vi "singleShot_defaultSetup.vi"() -> ()   [LabVIEW 2016]
uses:
  <userlib>/RSA_API/RSA_API.lvlib
panel:
  out "settings out":T1 {"window" items=["SpectrumWindow_Kaiser", "SpectrumWindow_Mil6dB", "SpectrumWindow_BlackmanHarris", "SpectrumWindow_Rectangle", "SpectrumWindow_FlatTop", "SpectrumWindow_Hann"]; "verticalUnit" items=["SpectrumVerticalUnit_dBm", "SpectrumVerticalUnit_Watt", "SpectrumVerticalUnit_Volt", "SpectrumVerticalUnit_Amp", "SpectrumVerticalUnit_dBmV"]}
  in  "Trace number":u32(ring) items=["SpectrumTrace1", "SpectrumTrace2", "SpectrumTrace3"]
  out "traceData out":sgl[](graph)
  out "outTracePoints out":i32
  out "Trace Ready":bool
  out "enable out":bool
  out "refLevel out":dbl
  out "cf out":dbl
  in  "deviceID":i32
  out "deviceType out":string
  out "deviceSerial out":string
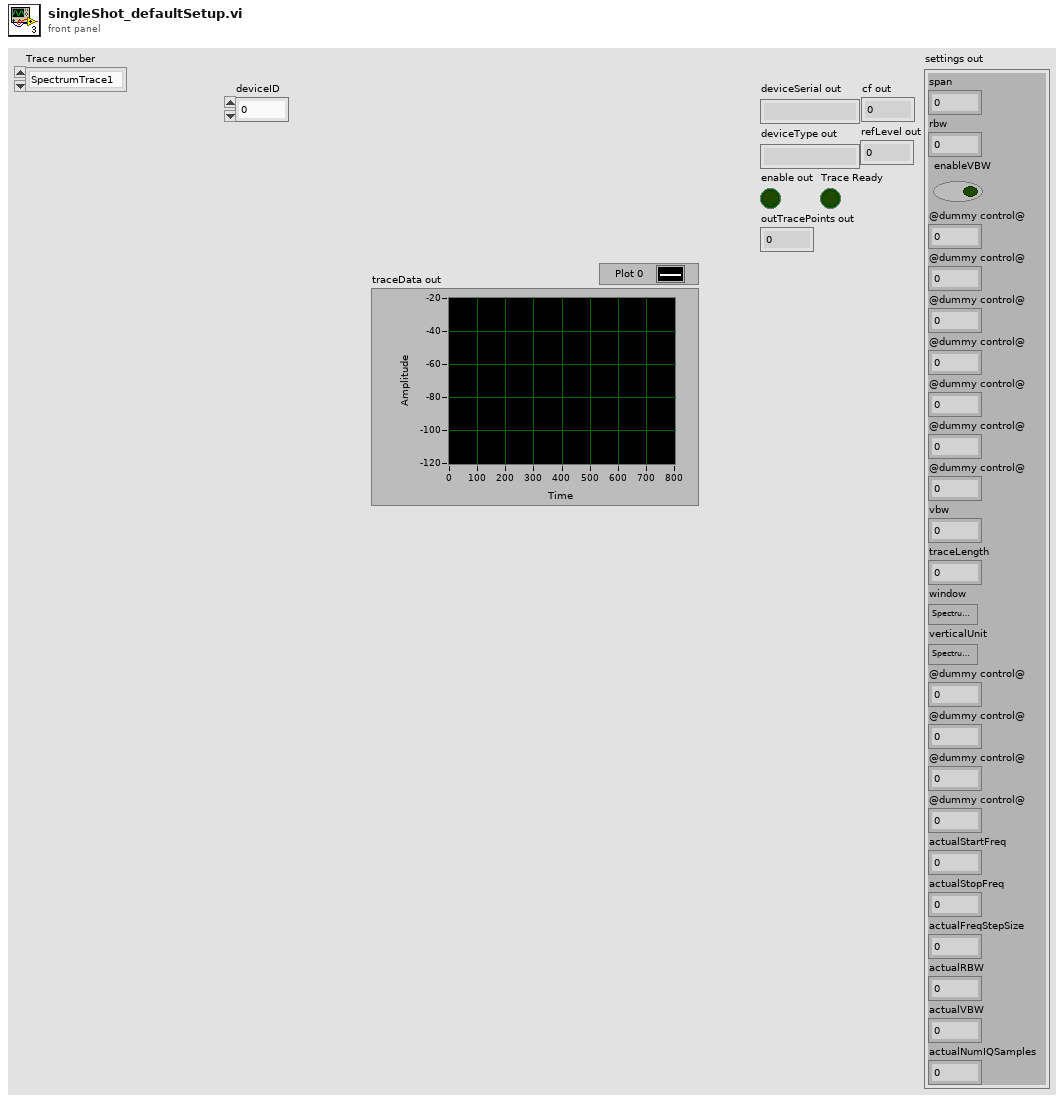
[diagram p1: front panel]
types:
  T1 = cluster{"span":dbl, "rbw":dbl, "enableVBW":bool, "@dummy control@":i8, "@dummy control@":i8, "@dummy control@":i8, "@dummy control@":i8, "@dummy control@":i8, "@dummy control@":i8, "@dummy control@":i8, "vbw":dbl, "traceLength":i32, "window":u32, "verticalUnit":u32, "@dummy control@":i8, "@dummy control@":i8, "@dummy control@":i8, "@dummy control@":i8, "actualStartFreq":dbl, "actualStopFreq":dbl, "actualFreqStepSize":dbl, "actualRBW":dbl, "actualVBW":dbl, "actualNumIQSamples":i32}
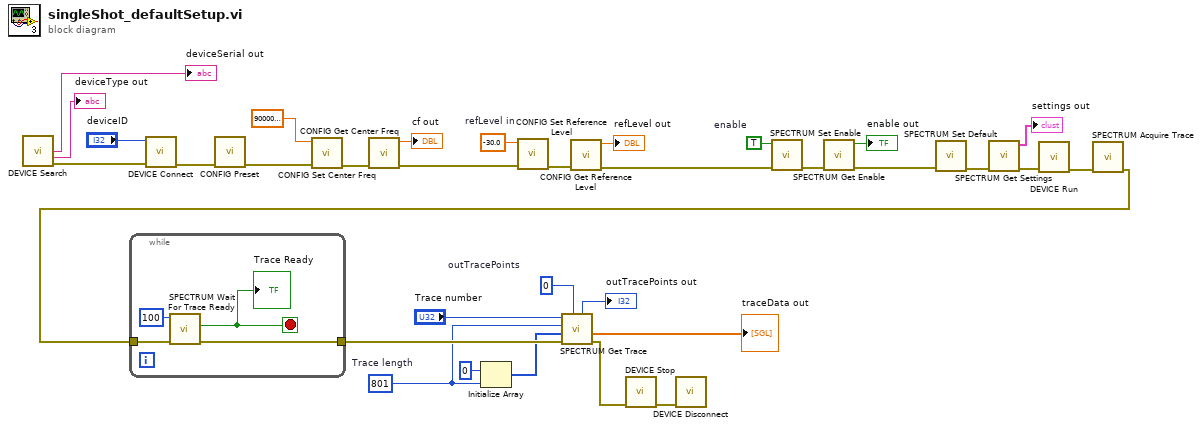
[diagram p0: block diagram]
diagram:
  w19 = TRUE  # enable
  w22 = -30.0  # refLevel in
  w10 = 801  # Trace length
  w11 = 0  # outTracePoints
  n1 = call <userlib>:"DEVICE Search.vi"() -> ("deviceSerial out"=→"deviceSerial out":string, "deviceType out"=→"deviceType out":string, "error out"=w30:errorcluster)  [unwired: 10 in, 3 out]
  n2 = call <userlib>:"DEVICE Connect.vi"("error in (no error)"=w30, "deviceID"="deviceID") -> ("error out"=w29:errorcluster)  [unwired: 8 in, 1 out]
  n3 = call <userlib>:"CONFIG Preset.vi"("error in (no error)"=w29) -> ("error out"=w28:errorcluster)  [unwired: 9 in, 1 out]
  n4 = call <userlib>:"CONFIG Set Center Freq.vi"("error in (no error)"=w28, "cf"=90000000.0) -> ("error out"=w27:errorcluster)  [unwired: 8 in, 1 out]
  n5 = call <userlib>:"CONFIG Get Center Freq.vi"("error in (no error)"=w27) -> ("error out"=w26:errorcluster, "cf out"=→"cf out":dbl)  [unwired: 8 in, 1 out]
  n6 = Initialize Array(0 ("element"), w10) -> (w8:i32[])
  n7 = call <userlib>:"CONFIG Set Reference Level.vi"("error in (no error)"=w26, "refLevel"=w22) -> ("error out"=w25:errorcluster)  [unwired: 8 in, 1 out]
  n8 = call <userlib>:"CONFIG Get Reference Level.vi"("error in (no error)"=w25) -> ("error out"=w20:errorcluster, "refLevel out"=→"refLevel out":dbl)  [unwired: 8 in, 1 out]
  n9 = call <userlib>:"SPECTRUM Set Enable.vi"("error in (no error)"=w20, "enable"=w19) -> ("error out"=w18:errorcluster)  [unwired: 8 in, 1 out]
  n10 = call <userlib>:"SPECTRUM Get Enable.vi"("error in (no error)"=w18) -> ("error out"=w16:errorcluster, "enable out"=→"enable out":bool)  [unwired: 8 in, 1 out]
  n11 = call <userlib>:"SPECTRUM Set Default.vi"("error in (no error)"=w16) -> ("error out"=w3:errorcluster)  [unwired: 9 in, 1 out]
  n12 = call <userlib>:"SPECTRUM Get Settings.vi"("error in (no error)"=w3) -> ("error out"=w2:errorcluster, "settings out"=→"settings out":T1)  [unwired: 8 in, 1 out]
  n13 = call <userlib>:"DEVICE Run.vi"("error in (no error)"=w2) -> ("error out"=w15:errorcluster)  [unwired: 9 in, 1 out]
  n14 = call <userlib>:"SPECTRUM Acquire Trace.vi"("error in (no error)"=w15) -> ("error out"=w14:errorcluster)  [unwired: 9 in, 1 out]
  n15 = while {
    tunnel: w14 -> [w35]
    tunnel: [w34] -> w13
    stop <- w36 stop-if-true
    n16 = call <userlib>:"SPECTRUM Wait For Trace Ready.vi"("error in (no error)"=w35, "timeoutMsec"=100) -> ("error out"=w34:errorcluster, "ready out"=w36:bool)  [unwired: 7 in, 1 out]
    "Trace Ready" <- w36
  }
  n17 = call <userlib>:"SPECTRUM Get Trace.vi"("outTracePoints"=w11, "error in (no error)"=w13, "traceData"=w8, "maxTracePoints"=w10, "trace"="Trace number") -> ("error out"=w5:errorcluster, "traceData out"=→"traceData out":sgl[], "outTracePoints out"=→"outTracePoints out":i32)  [unwired: 3 in, 1 out]
  n18 = call <userlib>:"DEVICE Stop.vi"("error in (no error)"=w5) -> ("error out"=w4:errorcluster)  [unwired: 9 in, 1 out]
  n19 = call <userlib>:"DEVICE Disconnect.vi"("error in (no error)"=w4) -> ()  [unwired: 9 in, 2 out]
